vi "Actor Core.vi"(8 "error in":errorcluster, 11 "DataProcessor in":refnum<class "DataProcessor.lvclass">) -> (0 "error out":errorcluster, 3 "Actor out":refnum<class "Actor.lvclass">)   [LabVIEW 2020, in "DataProcessor.lvlib" / "DataProcessor.lvclass"]
doc: "(<B>Filename</B>: Actor Framework.lvlib:Actor.lvclass:Actor Core.vi)\n\nReceives messages to the actor, reacts to them, and initiates any error handling that may shut the actor down.\n\nDescendant classes may override this VI to append parallel tasks for the actor to complete while it handles messages. Overrides use the Call Parent Class Method node."
uses:
  DataProcessor.lvclass
  <vilib>/ActorFramework/Actor/Actor.lvclass
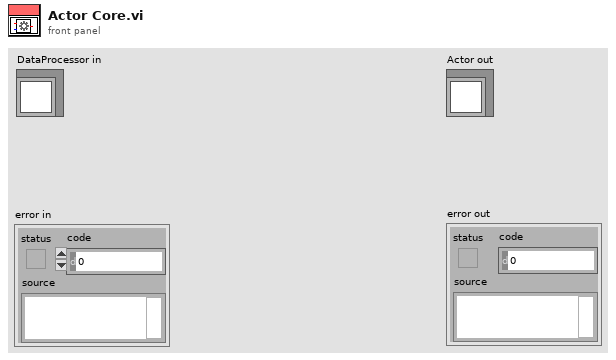
[diagram p1: front panel]
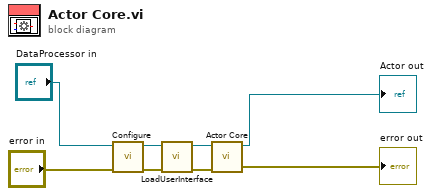
[diagram p0: block diagram]
diagram:
  n1 = call-dynamic "Configure.vi"("error in (no error)"="error in", "DataProcessor in"="DataProcessor in") -> ("error out"=w5:errorcluster, "DataProcessor out"=w2:refnum<class "DataProcessor.lvclass">)  [unwired: 8 in]
  n2 = call-dynamic "LoadUserInterface.vi"("error in (no error)"=w5, "DataProcessor in"=w2) -> ("error out"=w3:errorcluster, "DataProcessor out"=w1:refnum<class "DataProcessor.lvclass">)  [unwired: 8 in]
  n3 = call-parent "Actor Core.vi"("error in"=w3, "Actor in"=w1) -> ("error out"=→"error out":errorcluster, "Actor out"=→"Actor out":refnum<class "Actor.lvclass">)  [unwired: 8 in]
